vi "Parse Autonomous.vi"() -> ()   [LabVIEW 2012]
uses:
  Robot Global Data.vi
  Parse CSV From cRIO.vi
panel:
  out "Loop Time 2":u32(graph)
  out "Parsed Array":dbl[][](array[numeric])
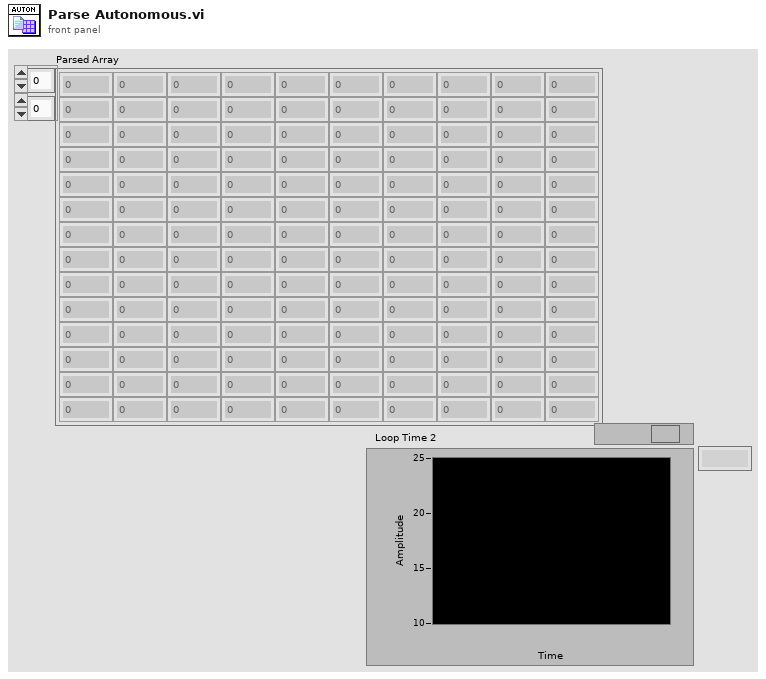
[diagram p1: front panel]
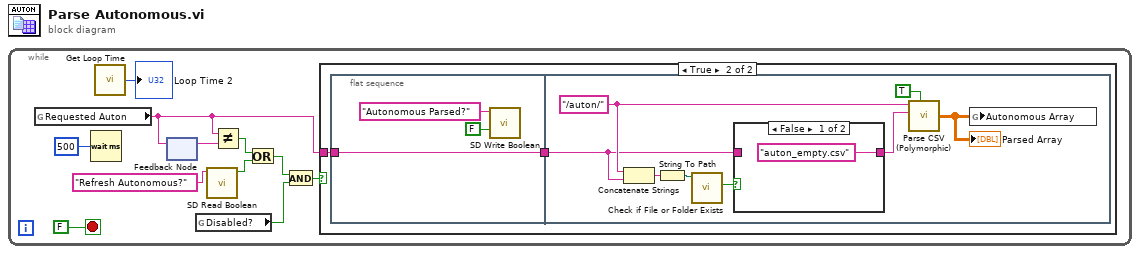
[diagram p0: block diagram]
diagram:
  n1 = while {
    stop <- FALSE stop-if-true
    n2 = global read "Robot Global Data.vi" "Requested Auton"() -> (w10:string)
    n3 = Wait (ms)(milliseconds to wait=u32 500) -> ()  [unwired: 1 out]
    n4 = call "Get Loop Time.vi"() -> ("Loop Time"=→"Loop Time 2":u32)  [unwired: 1 in]
    n5 = feedback-in #1(w10) -> ()
    n6 = feedback #1() -> (w9:string)  [unwired: 1 in]
    n7 = global read "Robot Global Data.vi" "Disabled?"() -> (w5:bool)
    n8 = call <vilib>:"SD Read Boolean.vi"("Name"="Refresh Autonomous?") -> ("Boolean"=w2:bool)  [unwired: 8 in, 2 out]
    n9 = Not Equal?(x=w10, y=w9) -> (x != y?=w6:bool)
    n10 = Or(x=w6, y=w2) -> (x .or. y?=w3:bool)
    n11 = And(x=w3, y=w5) -> (x .and. y?=w7:bool)
    n12 = case shown="True" w7 {
      tunnel: w10 -> [_ w13]
      frame False {
      }
      frame True {
        n13 = flat-sequence {
          tunnel: w13 -> [w16]
          tunnel: [w16] -> w12
          tunnel: w12 -> [w17]
          frame #0 {
            n14 = call <vilib>:"SD Write Boolean.vi"("Boolean"=FALSE, "Name"="Autonomous Parsed?") -> ()  [unwired: 8 in, 2 out]
          }
          frame #1 {
            w19 = "/auton/" ("string")
            n15 = Concatenate Strings(w19, w17) -> (w20:string)
            n16 = String To Path(string=w20) -> (path=w22:path)
            n17 = call <vilib>:"Check if File or Folder Exists.vi"("path"=w22) -> ("file or folder exists?"=w21:bool)  [unwired: 8 in, 2 out]
            n18 = case shown="False" w21 {
              tunnel: ["auton_empty.csv" ("string") w26] -> w24
              tunnel: w17 -> [_ w26]
              frame False {
              }
              frame True {
              }
            }
            n19 = call-poly "Parse CSV (Polymorphic).vi"("/path/"=w19, "File Name"=w24, "Header Row?"=TRUE) -> ("Output Array"=w18:dbl[][])  [unwired: 2 in]
            "Parsed Array" <- w18
            n20 = global write "Robot Global Data.vi" "Autonomous Array"(w18) -> ()
          }
        }
      }
    }
  }
